vi "TestRead.vi"() -> ()   [LabVIEW 2010]
panel:
  out "Bytes Read 2":u32
  out "Read Data 2":string
  out "FT_Status 2":u32(ring) items=["FT_OK", "FT_INVALID_HANDLE", "FT_DEVICE_NOT_FOUND", "FT_DEVICE_NOT_OPENED", "FT_IO_ERROR", "FT_INSUFFICIENT_RESOURCES", "FT_INVALID_PARAMETER", "FT_INVALID_BAUD_RATE", "FT_DEVICE_NOT_OPENED_FOR_ERASE", "FT_DEVICE_NOT_OPENED_FOR_WRITE", "FT_FAILED_TO_WRITE_DEVICE", "FT_EEPROM_READ_FAILED", "FT_EEPROM_WRITE_FAILED", "FT_EEPROM_ERASE_FAILED", "FT_EEPROM_NOT_PRESENT", "FT_EEPROM_NOT_PROGRAMMED", "FT_INVALID_ARGS", "FT_NOT_SUPPORTED", "FT_OTHER_ERROR"]
  out "Bytes Waiting 2":u32
  out "FT_Status":u32(ring) items=["FT_OK", "FT_INVALID_HANDLE", "FT_DEVICE_NOT_FOUND", "FT_DEVICE_NOT_OPENED", "FT_IO_ERROR", "FT_INSUFFICIENT_RESOURCES", "FT_INVALID_PARAMETER", "FT_INVALID_BAUD_RATE", "FT_DEVICE_NOT_OPENED_FOR_ERASE", "FT_DEVICE_NOT_OPENED_FOR_WRITE", "FT_FAILED_TO_WRITE_DEVICE", "FT_EEPROM_READ_FAILED", "FT_EEPROM_WRITE_FAILED", "FT_EEPROM_ERASE_FAILED", "FT_EEPROM_NOT_PRESENT", "FT_EEPROM_NOT_PROGRAMMED", "FT_INVALID_ARGS", "FT_NOT_SUPPORTED", "FT_OTHER_ERROR"]
  out "Read Data":string
  out "Bytes Read":u32
  out "Bytes Waiting":u32
  out "Status":bool
  out "Handle ChB 2":u32
  out "Handle ChA":u32
  out "Device Info List":T1(array[cluster]) {"FT_Handle" format="%.0x"; "LocID" format="%.0x"; "PID" format="%.0x"; "VID" format="%.0x"; "Type" items=["FT232B-FT245B", "FT8U232AM-FT8U245AM", "FT8U100AX", "UNKNOWN", "FT2232", "FT232R", "FT2232H", "FT4232H"]}
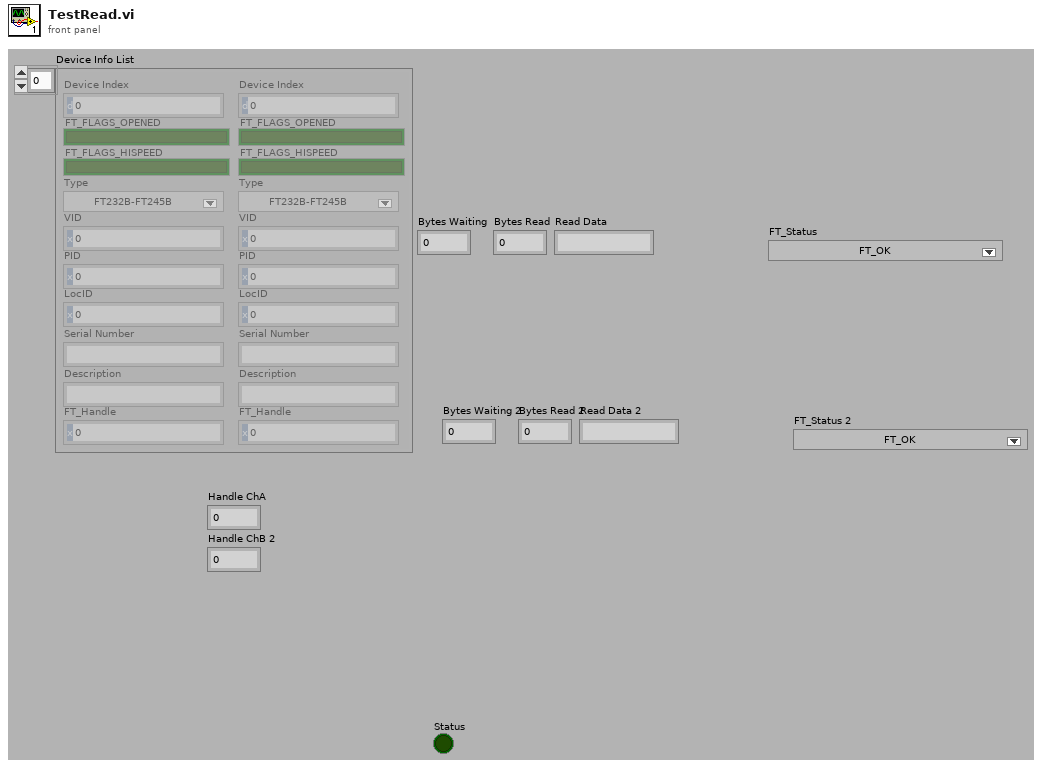
[diagram p1: front panel]
types:
  T1 = cluster{"Device Index":u32, "FT_FLAGS_OPENED":bool, "FT_FLAGS_HISPEED":bool, "Type":u32, "VID":u32, "PID":u32, "LocID":i32, "Serial Number":string, "Description":string, "FT_Handle":u32}[]
  T2 = cluster{"Device Index":u32, "FT_FLAGS_OPENED":bool, "FT_FLAGS_HISPEED":bool, "Type":u32, "VID":u32, "PID":u32, "LocID":i32, "Serial Number":string, "Description":string, "FT_Handle":u32}
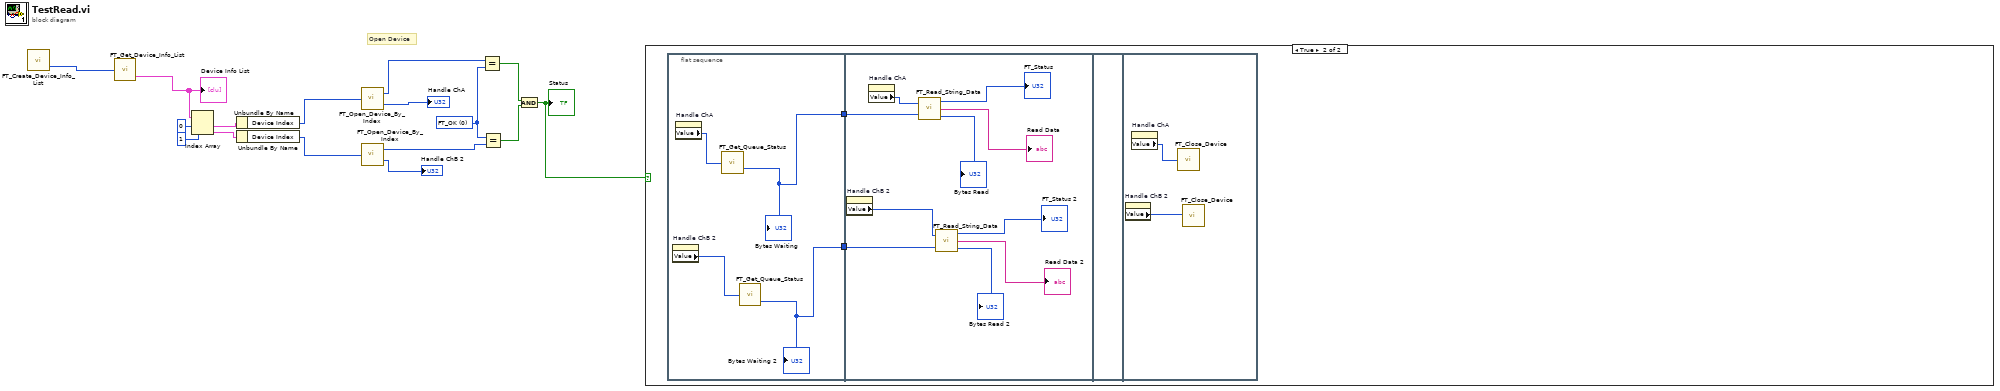
[diagram p0: block diagram]
diagram:
  w14 = u32 0 items=["FT_OK", "FT_INVALID_HANDLE", "FT_DEVICE_NOT_FOUND", "FT_DEVICE_NOT_OPENED", "FT_IO_ERROR", "FT_INSUFFICIENT_RESOURCES", "FT_INVALID_PARAMETER", "FT_INVALID_BAUD_RATE", "FT_DEVICE_NOT_OPENED_FOR_ERASE", "FT_DEVICE_NOT_OPENED_FOR_WRITE", "FT_FAILED_TO_WRITE_DEVICE", "FT_EEPROM_READ_FAILED", "FT_EEPROM_WRITE_FAILED", "FT_EEPROM_ERASE_FAILED", "FT_EEPROM_NOT_PRESENT", "FT_EEPROM_NOT_PROGRAMMED", "FT_INVALID_ARGS", "FT_NOT_SUPPORTED", "FT_OTHER_ERROR"] ("FT_Status")
  # "Open Device"
  n1 = call "FT_Create_Device_Info_List.vi"() -> ("Number of Devices"=w2:u32)  [unwired: 1 out]
  n2 = call "FT_Get_Device_Info_List.vi"("Number Of Devices"=w2) -> ("Device Info List"=w3:T1)  [unwired: 1 out]
  "Device Info List" <- w3
  n3 = Index Array(array=w3, index #1=0 ("index"), index #2=1 ("index")) -> (element #1=w4:T2, element #2=w7:T2)
  n4 = Unbundle By Name(w4) -> ("Device Index"=w8:u32)
  n5 = Unbundle By Name(w7) -> ("Device Index"=w9:u32)
  n6 = call "FT_Open_Device_By_Index.vi"("Device Index"=w8) -> ("FT_Status"=w12:u32, "Handle"=→"Handle ChA":u32)
  n7 = call "FT_Open_Device_By_Index.vi"("Device Index"=w9) -> ("FT_Status"=w13:u32, "Handle"=→"Handle ChB 2":u32)
  n8 = Equal?(x=w12, y=w14) -> (x = y?=w15:bool)
  n9 = Equal?(x=w14, y=w13) -> (x = y?=w16:bool)
  n10 = And(x=w15, y=w16) -> (x .and. y?=w1:bool)
  "Status" <- w1
  n11 = case shown="True" w1 {
    frame False {
    }
    frame True {
      n12 = flat-sequence {
        tunnel: [w21] -> w18
        tunnel: [w20] -> w17
        tunnel: w18 -> [w31]
        tunnel: w17 -> [w24]
        frame #0 {
          n13 = property on="Handle ChB 2" class="DigNum (strict)"() -> ("Value"=w19:u32)  [unwired: 2 in, 2 out]
          n14 = property on="Handle ChA" class="DigNum (strict)"() -> ("Value"=w22:u32)  [unwired: 2 in, 2 out]
          n15 = call "FT_Get_Queue_Status.vi"("Handle"=w22) -> ("Bytes Waiting"=w21:u32)  [unwired: 1 out]
          "Bytes Waiting" <- w21
          n16 = call "FT_Get_Queue_Status.vi"("Handle"=w19) -> ("Bytes Waiting"=w20:u32)  [unwired: 1 out]
          "Bytes Waiting 2" <- w20
        }
        frame #1 {
          n17 = property on="Handle ChB 2" class="DigNum (strict)"() -> ("Value"=w23:u32)  [unwired: 2 in, 2 out]
          n18 = property on="Handle ChA" class="DigNum (strict)"() -> ("Value"=w32:u32)  [unwired: 2 in, 2 out]
          n19 = call "FT_Read_String_Data.vi"("Handle"=w32, "Bytes To Read"=w31) -> ("FT_Status"=→"FT_Status":u32, "Read Data"=→"Read Data":string, "Bytes Read"=→"Bytes Read":u32)
          n20 = call "FT_Read_String_Data.vi"("Handle"=w23, "Bytes To Read"=w24) -> ("FT_Status"=→"FT_Status 2":u32, "Read Data"=→"Read Data 2":string, "Bytes Read"=→"Bytes Read 2":u32)
        }
        frame #2 {
        }
        frame #3 {
          n21 = property on="Handle ChB 2" class="DigNum (strict)"() -> ("Value"=w34:u32)  [unwired: 2 in, 2 out]
          n22 = property on="Handle ChA" class="DigNum (strict)"() -> ("Value"=w33:u32)  [unwired: 2 in, 2 out]
          n23 = call "FT_Close_Device.vi"("Handle"=w33) -> ()  [unwired: 1 out]
          n24 = call "FT_Close_Device.vi"("Handle"=w34) -> ()  [unwired: 1 out]
        }
      }
    }
  }
